vi "PID Relay Auto Tune.vi"(0 "Setpoint in":dbl(slide)=30.8641975308642 scale=0.0..100.0 scale format="%.1f", 1 "Calculate Parameters":bool, 2 "Relay Setpoint":bool, 3 "autotuning parameters":T2={"controller type"=1, "relay cycles"=3, "relay amplitude"=1.0, "control specification"=2, "PV noise level"=0.1} {"PV noise level" format="%.2f"; "control specification" items=["normal", "fast", "slow"]; "relay amplitude" format="%.2f"; "controller type" items=["PID", "PI", "P"]}, 5 "Process Variable":dbl(slide)=19.583333333333336 scale=0.0..100.0 scale format="%.1f", 9 "PID gains":T1={"proportional gain (Kc)"=1.0, "integral time (Ti, min)"=0.01, "derivative time (Td, min)"=0.0} {"derivative time (Td, min)" format="%.3f"; "integral time (Ti, min)" format="%.3f"; "proportional gain (Kc)" format="%.3f"}, 11 "dt (s)":dbl=-1.0 format="%.3f", 12 "reinitialize? (F)":bool) -> (4 "setpoint out":dbl(slide)=30.8641975308642 scale=0.0..100.0 scale format="%.1f", 6 "tuning completed?":bool, 10 "tuned PID gains":T1={"proportional gain (Kc)"=1.0, "integral time (Ti, min)"=0.01, "derivative time (Td, min)"=0.0} {"derivative time (Td, min)" format="%.3f"; "integral time (Ti, min)" format="%.3f"; "proportional gain (Kc)" format="%.3f"})   [LabVIEW 2017, in "NI_PID_autopid.lvlib"]
doc: "This VI performs the setpoint relay experiment for the autotuning procedure."
uses:
  <vilib>/addons/control/pid/NI_PID_autopid.lvlib
panel:
  # "Relay Auto Tune"
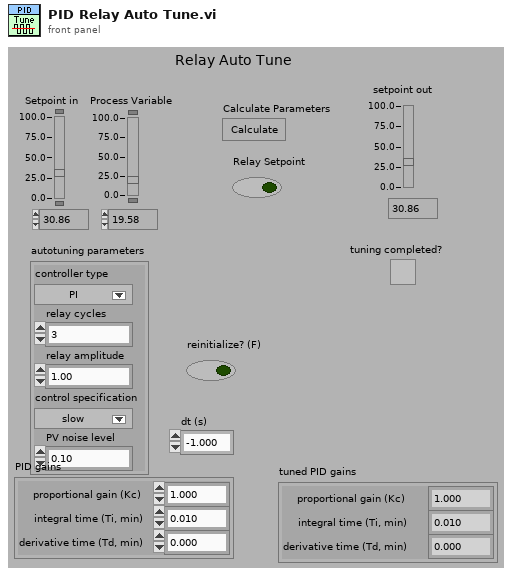
[diagram p1: front panel]
types:
  T1 = cluster{"proportional gain (Kc)":dbl, "integral time (Ti, min)":dbl, "derivative time (Td, min)":dbl}
  T2 = cluster{"controller type":u16, "relay cycles":i32, "relay amplitude":dbl, "control specification":u16, "PV noise level":dbl}
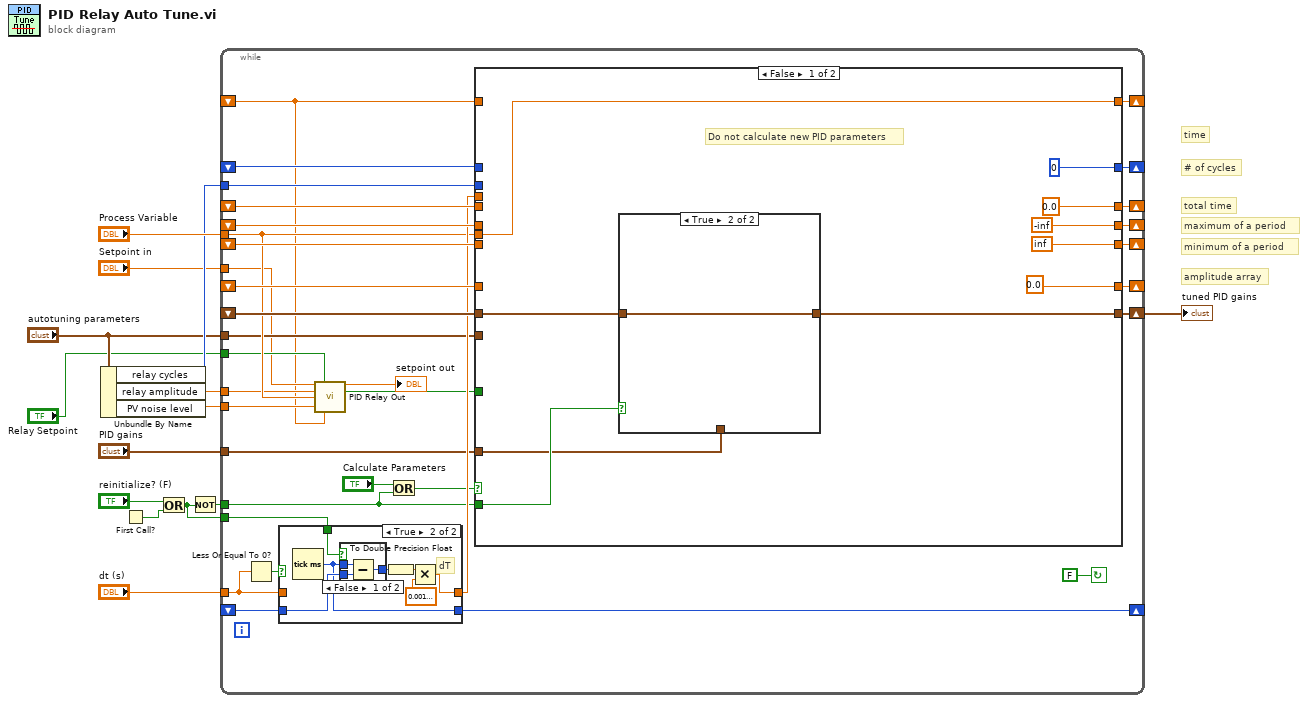
[diagram p0: block diagram]
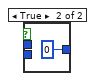
[diagram p3: hidden frame]
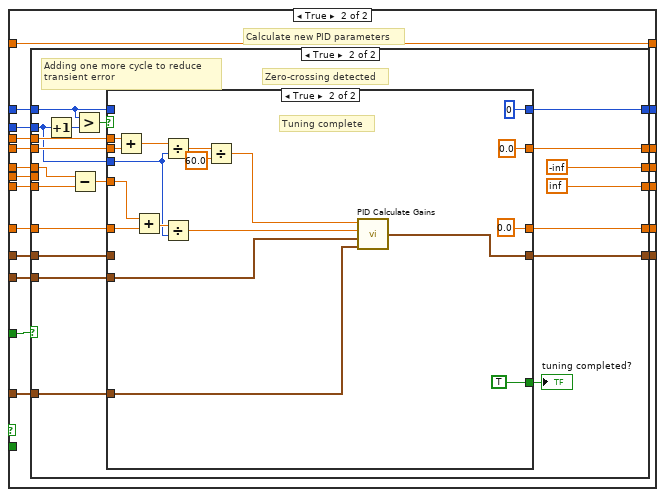
[diagram p5: hidden frame]
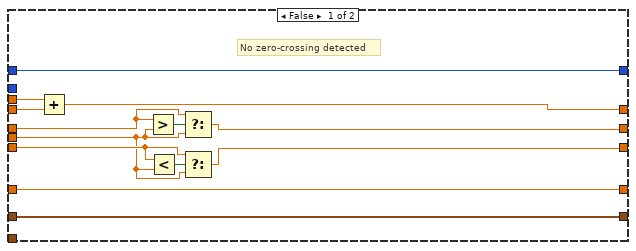
[diagram p6: hidden frame]
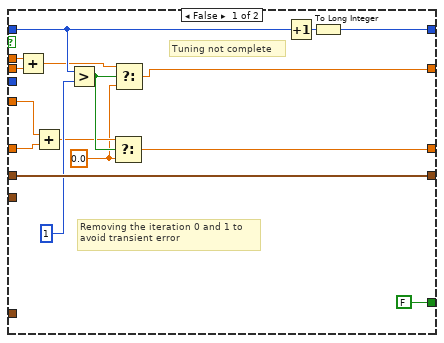
[diagram p7: hidden frame]
diagram:
  # "time"
  # "amplitude array"
  # "total time"
  # "minimum of a period"
  # "maximum of a period"
  # "# of cycles"
  n1 = Unbundle By Name("autotuning parameters") -> ("relay cycles"=w8:i32, "relay amplitude"=w4:dbl, "PV noise level"=w3:dbl)
  n2 = First Call?() -> (First Call?: T/F=w10:bool)
  n3 = Or(x="reinitialize? (F)", y=w10) -> (x .or. y?=w2:bool)
  n4 = Not(x=w2) -> (.not. x?=w13:bool)
  n5 = while {
    shift-left: _ -> [w38]
    shift-right: [w37] -> _
    shift-left: _ -> [w33]
    shift-right: [w32] -> _
    shift-left: _ -> [w40]
    shift-right: [w35] -> w14
    shift-left: _ -> [w43]
    shift-right: [w44] -> _
    shift-left: _ -> [w42]
    shift-right: [w45] -> _
    shift-left: _ -> [w46]
    shift-right: [w47] -> _
    shift-left: _ -> [w41]
    shift-right: [w48] -> _
    tunnel: w2 -> [w30]
    tunnel: w13 -> [w27]
    tunnel: "dt (s)" -> [w26]
    tunnel: "Process Variable" -> [w25]
    tunnel: w8 -> [w24]
    tunnel: w3 -> [w23]
    tunnel: w4 -> [w22]
    tunnel: "autotuning parameters" -> [w21]
    tunnel: "PID gains" -> [w20]
    tunnel: "Setpoint in" -> [w17]
    tunnel: "Relay Setpoint" -> [w19]
    shift-right: [w16] -> _
    shift-left: _ -> [w15]
    stop <- FALSE continue-if-true
    n6 = Less Or Equal To 0?(x=w26) -> (x <= 0?=w34:bool)
    n7 = case shown="True" w34 {
      tunnel: [w50 w54] -> w31
      tunnel: w33 -> [w49 w53]
      tunnel: [w49 w52] -> w32
      tunnel: w26 -> [w50 _]
      tunnel: w30 -> [_ w51]
      frame False {
      }
      frame True {
        # "dT"
        n8 = Tick Count (ms)() -> (millisecond timer value=w52:u32)
        n9 = case shown="False" w51 {
          tunnel: [w60 u32 0] -> w56
          tunnel: w53 -> [w59 _]
          tunnel: w52 -> [w58 _]
          frame False {
            n10 = Subtract(x=w58, y=w59) -> (x-y=w60:u32)
          }
          frame True {
          }
        }
        n11 = To Double Precision Float(number=w56) -> (double precision float=w55:dbl)
        n12 = Multiply(x=w55, y=0.0010000000474974513) -> (x*y=w54:dbl)
      }
    }
    n13 = call <vilib>:"PID Relay Out.vi"("Setpoint Reference"=w17, "Relay Setpoint"=w19, "Relay Amplitude"=w22, "Process Variable"=w25, "Noise Disturbance"=w23, "Process Variable Reference"=w15) -> ("relay output"=→"setpoint out":dbl, "Zero Crossing"=w18:bool)  [unwired: 2 in, 6 out]
    n14 = Or(x="Calculate Parameters", y=w27) -> (x .or. y?=w28:bool)
    n15 = case shown="False" w28 {
      tunnel: w41 -> [_ w80]
      tunnel: [0 w81] -> w48
      tunnel: [-inf w82] -> w47
      tunnel: w46 -> [_ w92]
      tunnel: w42 -> [_ w91]
      tunnel: [0.0 w84] -> w45
      tunnel: [inf w83] -> w44
      tunnel: w43 -> [_ w85]
      tunnel: w24 -> [_ w89]
      tunnel: [w66 w86] -> w35
      tunnel: w40 -> [w67 w90]
      tunnel: w18 -> [_ w88]
      tunnel: w31 -> [_ w87]
      tunnel: w38 -> [_ w79]
      tunnel: [0.0 ("f") w78] -> w37
      tunnel: w21 -> [_ w77]
      tunnel: w20 -> [w64 w76]
      tunnel: w27 -> [w65 _]
      tunnel: w25 -> [w62 w75]
      tunnel: [w62 w74] -> w16
      tunnel: w15 -> [_ w74]
      frame False {
        # "Do not calculate new PID parameters"
        n16 = case shown="True" w65 {
          tunnel: [w72 w73] -> w66
          tunnel: w67 -> [_ w73]
          tunnel: w64 -> [w72 _]
          frame False {
          }
          frame True {
          }
        }
      }
      frame True {
        # "Calculate new PID parameters"
        n17 = case shown="True" w88 {
          tunnel: w80 -> [w105 w112]
          tunnel: [w105 w114] -> w81
          tunnel: [w104 -inf] -> w82
          tunnel: w92 -> [w103 w125]
          tunnel: w91 -> [w102 w123]
          tunnel: [w102 w121] -> w84
          tunnel: [w99 inf] -> w83
          tunnel: w85 -> [w100 w124]
          tunnel: w89 -> [_ w109]
          tunnel: w90 -> [w97 w120]
          tunnel: w87 -> [w95 w119]
          tunnel: [w97 w118] -> w86
          tunnel: w79 -> [w96 w111]
          tunnel: [w94 w110] -> w78
          tunnel: w77 -> [_ w108]
          tunnel: w76 -> [_ w107]
          tunnel: w75 -> [w93 _]
          frame False {
            # "No zero-crossing detected"
            n18 = Add(x=w95, y=w96) -> (x+y=w94:dbl)
            n19 = Greater?(x=w103, y=w93) -> (0:w98:bool)
            n20 = Less?(x=w100, y=w93) -> (x < y?=w101:bool)
            n21 = Select(t=w103, s=w98, f=w93) -> (s? t:f=w104:dbl)
            n22 = Select(t=w100, s=w101, f=w93) -> (s? t:f=w99:dbl)
          }
          frame True {
            # "Adding one more cycle to reduce\ntransient error"
            # "Zero-crossing detected"
            n23 = Increment(x=w109) -> (x+1=w106:i32)
            n24 = Subtract(x=w125, y=w124) -> (x-y=w122:dbl)
            n25 = Greater?(x=w112, y=w106) -> (0:w113:bool)
            n26 = case shown="True" w113 {
              tunnel: w123 -> [w133 w146]
              tunnel: w122 -> [w134 w147]
              tunnel: [w128 0.0] -> w121
              tunnel: [w139 0] -> w114
              tunnel: w112 -> [w132 _]
              tunnel: [FALSE TRUE] -> w117
              tunnel: [w141 w142] -> w118
              tunnel: w120 -> [w141 _]
              tunnel: w119 -> [w138 w154]
              tunnel: w111 -> [w137 w155]
              tunnel: [w136 0.0 ("f")] -> w110
              tunnel: w109 -> [_ w144]
              tunnel: w108 -> [_ w151]
              tunnel: w107 -> [_ w149]
              frame False {
                w127 = 0.0 ("f")
                # "Removing the iteration 0 and 1 to \navoid transient error"
                # "Tuning not complete"
                n27 = Add(x=w138, y=w137) -> (x+y=w126:dbl)
                n28 = Add(x=w134, y=w133) -> (x+y=w129:dbl)
                n29 = Greater?(x=w132, y=1) -> (0:w130:bool)
                n30 = Select(t=w129, s=w130, f=w127) -> (s? t:f=w128:dbl)
                n31 = Select(t=w126, s=w130, f=w127) -> (s? t:f=w136:dbl)
                n32 = Increment(x=w132) -> (x+1=w140:i32)
                n33 = To Long Integer(number=w140) -> (32bit integer=w139:i32)
              }
              frame True {
                # "Tuning complete"
                n34 = Add(x=w154, y=w155) -> (x+y=w153:dbl)
                n35 = Add(x=w147, y=w146) -> (x+y=w145:dbl)
                n36 = Divide(x=w153, y=w144) -> (x/y=w152:dbl)
                n37 = Divide(x=w145, y=w144) -> (x/y=w143:dbl)
                n38 = Divide(x=w152, y=60.0) -> (x/y=w150:dbl)
                n39 = call <vilib>:"PID Calculate Gains.vi"("PID parameters"=w149, "autotuning parameters"=w151, "Mean amplitude"=w143, "Mean period"=w150) -> ("tuned PID parameters"=w142:cluster{"Kc":dbl, "Ti":dbl, "Td":dbl})  [unwired: 2 out]
              }
            }
            "tuning completed?" <- w117
          }
        }
      }
    }
  }
  "tuned PID gains" <- w14
